vi "CMN_Str2Decimal.vi"(8 "error in (no error)":errorcluster, 10 "number in":string) -> (0 "error out":errorcluster, 2 "decimal number":dbl)   [LabVIEW 2016]
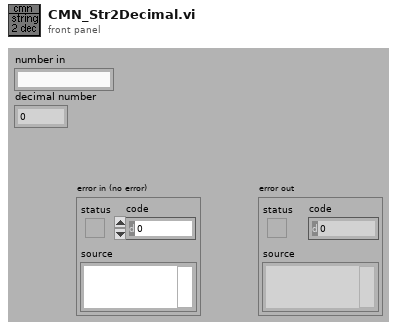
[diagram p1: front panel]
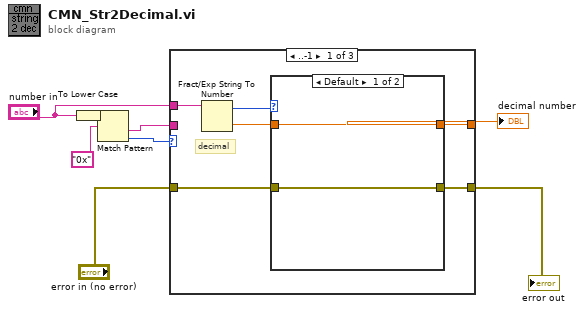
[diagram p0: block diagram]
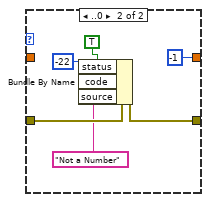
[diagram p2: hidden frame]
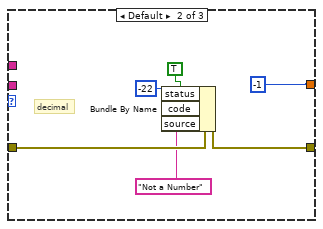
[diagram p3: hidden frame]
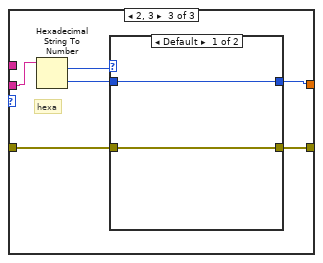
[diagram p4: hidden frame]
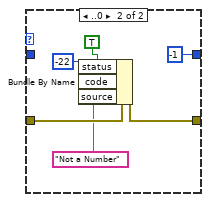
[diagram p5: hidden frame]
diagram:
  n1 = To Lower Case(string="number in") -> (all lower case string=w1:string)
  n2 = Match Pattern(string=w1, regular expression="0x") -> (after substring=w6:string, offset past match=w7:i32)  [unwired: 3 out]
  n3 = case shown="..-1" w7 {
    tunnel: [w9 -1 w29] -> w5
    tunnel: w6 -> [_ _ w31]
    tunnel: "error in (no error)" -> [w13 w28 w34]
    tunnel: [w12 w27 w33] -> w3
    tunnel: "number in" -> [w11 _ _]
    frame ..-1 {
      # "decimal"
      n4 = Fract/Exp String To Number(string=w11) -> (offset past number=w14:i32, number=w10:dbl)  [unwired: 3 out]
      n5 = case shown="Default" w14 {
        tunnel: w13 -> [w16 w22]
        tunnel: [w16 w21] -> w12
        tunnel: w10 -> [w15 _]
        tunnel: [w15 -1] -> w9
        frame Default {
        }
        frame ..0 {
          n6 = Bundle By Name(cluster=w22, "status"=TRUE, "code"=-22, "source"="Not a Number") -> (w21:errorcluster)
        }
      }
    }
    frame Default {
      # "decimal"
      n7 = Bundle By Name(cluster=w28, "status"=TRUE, "code"=-22, "source"="Not a Number") -> (w27:errorcluster)
    }
    frame 2, 3 {
      # "hexa"
      n8 = Hexadecimal String To Number(string=w31) -> (offset past number=w32:i32, number=w30:u32)  [unwired: 2 out]
      n9 = case shown="Default" w32 {
        tunnel: w34 -> [w36 w42]
        tunnel: [w36 w41] -> w33
        tunnel: w30 -> [w35 _]
        tunnel: [w35 -1] -> w29
        frame Default {
        }
        frame ..0 {
          n10 = Bundle By Name(cluster=w42, "status"=TRUE, "code"=-22, "source"="Not a Number") -> (w41:errorcluster)
        }
      }
    }
  }
  "decimal number" <- w5
  "error out" <- w3
